vi "wait.vi"(1 "State to wait for":i32, 2 "Waiting Loop ID":i32, 3 "Time (ms)":i32, 4 "Current Loop ID":i32) -> (0 "Done?":bool)   [LabVIEW 2013]
doc: "This VI allows you to wait for a specified amount of time before advancing, or for a different subsystem to reach a different state. Useful in autonomous applications."
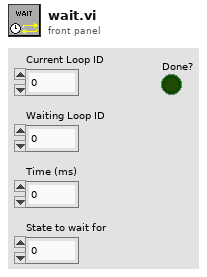
[diagram p1: front panel]
types:
  T1 = typedef "subStates.ctl" = enum16{"null", "wait", "driver control", "auto", "manual override", "hold position", "rotate", "test", "end"}
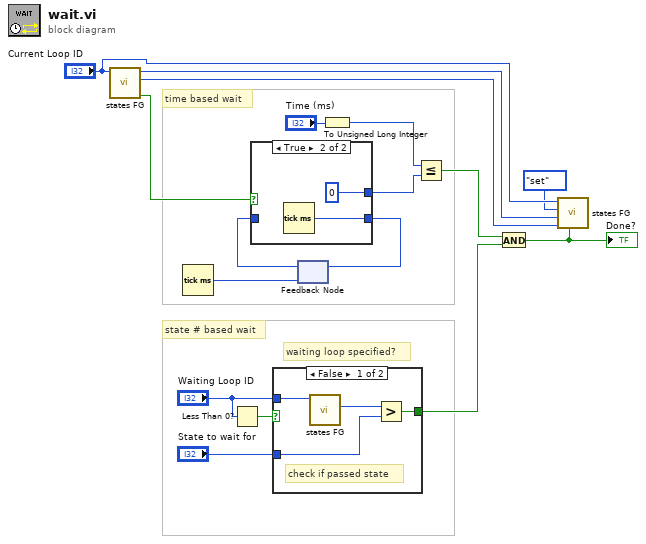
[diagram p0: block diagram]
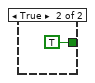
[diagram p2: hidden frame]
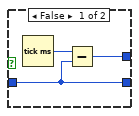
[diagram p3: hidden frame]
diagram:
  # "state # based wait"
  # "time based wait"
  # "waiting loop specified?"
  n1 = call "states FG.vi"("Loop ID"="Current Loop ID") -> ("first call?"=w17:bool, "state # out"=w9:i32, "subState out"=w10:T1)  [unwired: 7 in, 1 out]
  n2 = Tick Count (ms)() -> (millisecond timer value=w4:u32)
  n3 = Less Than 0?(x="Waiting Loop ID") -> (x < 0?=w5:bool)
  n4 = case shown="False" w5 {
    tunnel: "Waiting Loop ID" -> [w21 _]
    tunnel: "State to wait for" -> [w20 _]
    tunnel: [w19 TRUE] -> w12
    frame False {
      # "check if passed state"
      n5 = call "states FG.vi"("Loop ID"=w21) -> ("state # out"=w18:i32)  [unwired: 7 in, 3 out]
      n6 = Greater?(x=w18, y=w20) -> (0:w19:bool)
    }
    frame True {
    }
  }
  n7 = feedback #1(w4) -> (w15:u32)
  n8 = case shown="True" w17 {
    tunnel: [w24 w27] -> w16
    tunnel: w15 -> [w24 _]
    tunnel: [w23 u32 0] -> w14
    frame False {
      n9 = Tick Count (ms)() -> (millisecond timer value=w25:u32)
      n10 = Subtract(x=w25, y=w24) -> (x-y=w23:u32)
    }
    frame True {
      n11 = Tick Count (ms)() -> (millisecond timer value=w27:u32)
    }
  }
  n12 = feedback-in #1(w16) -> ()
  n13 = To Unsigned Long Integer(number="Time (ms)") -> (unsigned 32bit integer=w7:u32)
  n14 = Less Or Equal?(x=w7, y=w14) -> (x <= y?=w3:bool)
  n15 = And(x=w3, y=w12) -> (x .and. y?=w11:bool)
  "Done?" <- w11
  n16 = call "states FG.vi"("exit in"=w11, "state # in"=w9, "subState in"=w10, "menu (get)"=enum16{"set", "get"}."set", "Loop ID"="Current Loop ID") -> ()  [unwired: 3 in, 4 out]
